vi "Heat1D_Solver.vi"(0 "F(t, x)":dbl[][](array[numeric]), 1 "Initial Value":dbl[](array[numeric]), 5 "k":dbl=1.0, 7 "a":dbl, 9 "Domain":T1={"t"={"initial t"=0.0, "final t"=1.0, "# of t-points"=11}, "x"={"start x"=0.0, "end x"=1.0, "# of x-points"=11}}, 11 "error in (no error)":errorcluster, 12 "Boundary Condition":cluster{"type":T2, "Value":dbl[]}[](array[cluster]) {"type" items=["Dirichlet", "Neumann"]}) -> (4 "U(t, x)":dbl[][](array[numeric]), 15 "error out":errorcluster)   [LabVIEW 2020, in "NI_PDE.lvlib"]
uses:
  <vilib>/gmath/NI_PDE.lvlib
  <vilib>/gmath/pde.llb/Common/PDE_BC Type.ctl
  <vilib>/Analysis/NI_AALPro.lvlib
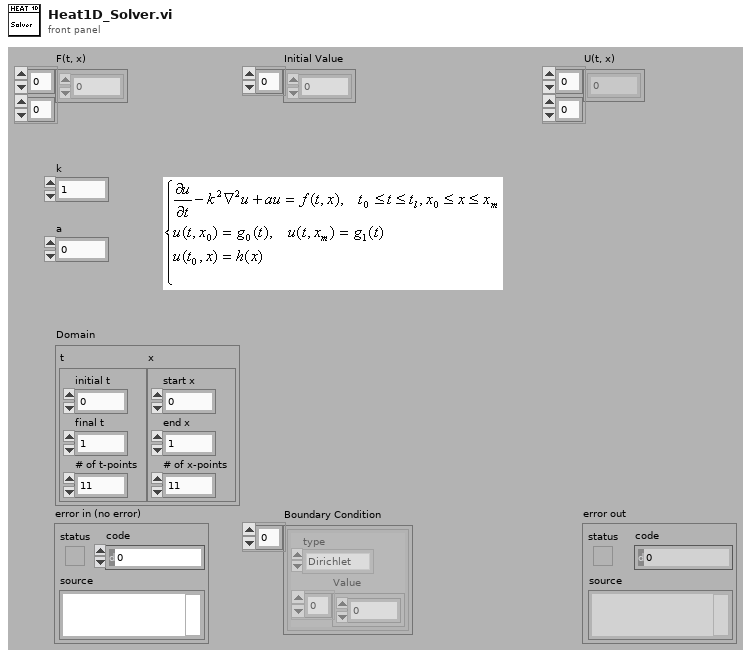
[diagram p1: front panel]
types:
  T1 = cluster{"t":cluster{"initial t":dbl, "final t":dbl, "# of t-points":i32}, "x":cluster{"start x":dbl, "end x":dbl, "# of x-points":i32}}
  T2 = typedef "NI_PDE.lvlib/PDE_BC Type.ctl" = i32
  T3 = cluster{"initial t":dbl, "final t":dbl, "# of t-points":i32}
  T4 = cluster{"Diagonal":dbl[], "Super Diagonal":dbl[], "2nd Super Diagonal":dbl[]}
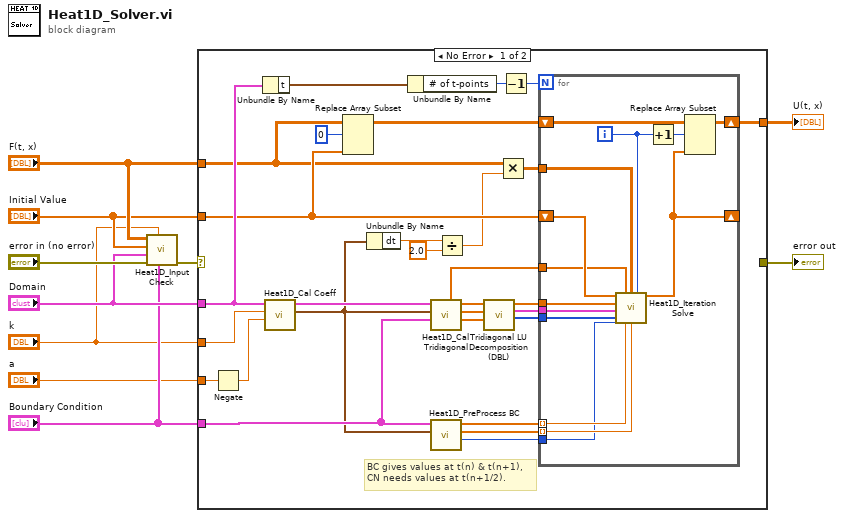
[diagram p0: block diagram]
diagram:
  n1 = call <vilib>:"Heat1D_Input Check.vi"("Boundary Condition"="Boundary Condition", "k"="k", "error in (no error)"="error in (no error)", "Domain"="Domain", "Initial Value"="Initial Value", "F(t, x)"="F(t, x)") -> ("error out"=w10:errorcluster)  [unwired: 5 out]
  n2 = case shown="No Error" w10 {
    selector: w10 -> [_ w54]
    tunnel: "F(t, x)" -> [w17 _]
    tunnel: "Domain" -> [w37 _]
    tunnel: "k" -> [w25 _]
    tunnel: "Initial Value" -> [w23 _]
    tunnel: "a" -> [w28 _]
    tunnel: "Boundary Condition" -> [w27 _]
    tunnel: [_ w54] -> w4
    tunnel: [w21 _] -> w3
    frame No Error {
      # "BC gives values at t(n) & t(n+1),\nCN needs values at t(n+1/2)."
      n3 = Negate(x=w28) -> (-x=w26:dbl)
      n4 = Unbundle By Name(w37) -> ("t"=w20:T3)
      n5 = call <vilib>:"Heat1D_Cal Coeff.vi"("a"=w26, "k"=w25, "Domain"=w37) -> ("Coefficients"=w14:cluster{"r":dbl, "s":dbl, "dt":dbl, "dx":dbl}, "Domain Dup"=w15:T1)  [unwired: 7 out]
      n6 = Replace Array Subset(array=w17, new element=w23, index (row)=0) -> (w22:dbl[][])  [unwired: 1 in]
      n7 = Unbundle By Name(w14) -> ("dt"=w13:dbl)
      n8 = Unbundle By Name(w20) -> ("# of t-points"=w18:i32)
      n9 = call <vilib>:"Heat1D_Cal Tridiagonal.vi"("Boundary Condition"=w27, "Coefficients"=w14, "Domain"=w15) -> ("Super Diagonal"=w34:dbl[], "Main Diagonal"=w35:dbl[], "Sub Diagonal"=w36:dbl[], "Coeff Array"=w30:dbl[])  [unwired: 2 in, 3 out]
      n10 = call <vilib>:"Heat1D_PreProcess BC.vi"("Coefficients"=w14, "Boundary Condition"=w27) -> ("BC Type"=w29:i32, "Right BC out"=w38:dbl[], "Left BC out"=w39:dbl[])  [unwired: 1 in, 6 out]
      n11 = Divide(x=w13, y=2.0 ("value")) -> (x/y=w11:dbl)
      n12 = call <vilib>:"Tridiagonal LU Decomposition (DBL).vi"("Super Diagonal"=w34, "Diagonal"=w35, "Sub Diagonal"=w36) -> ("Pivot"=w31:i32[], "U"=w32:T4, "L"=w33:dbl[])  [unwired: 6 out]
      n13 = Multiply(x=w17, y=w11) -> (x*y=w16:dbl[][])
      n14 = Decrement(x=w18) -> (x-1=w19:i32)
      n15 = for {
        N: w19 -> [_]
        tunnel: w30 -> [w52]
        tunnel: w16 -> [w51]
        shift-right: [w41] -> _
        shift-left: w23 -> [w53]
        tunnel: w39 -> [w50] mode=indexing
        tunnel: w38 -> [w49] mode=indexing
        tunnel: w33 -> [w48]
        tunnel: w32 -> [w47]
        tunnel: w31 -> [w46]
        tunnel: w29 -> [w45]
        shift-right: [w42] -> w21
        shift-left: w22 -> [w44]
        i -> [w40]
        n16 = call <vilib>:"Heat1D_Iteration Solve.vi"("U(n)"=w53, "Coeff Array"=w52, "F(x,t)"=w51, "step"=w40, "L"=w48, "U"=w47, "Pivot"=w46, "BC Type"=w45, "Left BC"=w50, "Right BC"=w49) -> ("U(n+1)"=w41:dbl[])  [unwired: 5 out]
        n17 = Increment(x=w40) -> (x+1=w43:i32)
        n18 = Replace Array Subset(array=w44, new element=w41, index (row)=w43) -> (w42:dbl[][])  [unwired: 1 in]
      }
    }
    frame Error {
    }
  }
  "U(t, x)" <- w3
  "error out" <- w4
